vi "WriteEvtSignal.vi"(8 "error in (no error)":errorcluster, 10 "EvtSignal":dbl[][](array[numeric]), 11 "Simulation in":refnum<class "Simulation.lvclass">) -> (0 "error out":errorcluster, 3 "Simulation out":refnum<class "Simulation.lvclass">)   [LabVIEW 2014, in "SamplerPlugins.lvlib" / "Simulation.lvclass"]
uses:
  Simulation.lvclass
  Simulation.lvclass/Simulation.ctl
  Accessors/Write EvtSignalArray.vi
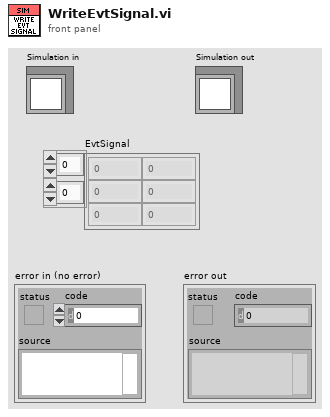
[diagram p1: front panel]
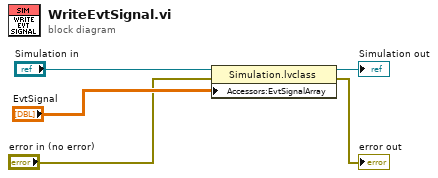
[diagram p0: block diagram]
diagram:
  n1 = property class="Simulation.lvclass"(reference="Simulation in", error in="error in (no error)", "Accessors:EvtSignalArray"="EvtSignal") -> (reference out=→"Simulation out":refnum<class "Simulation.lvclass">, error out=→"error out":errorcluster)
